vi "pp2_util_paintTableElement.vi"(9 "Color Box":u32(colorbox)=16448250, 10 "Numeric":i32, 11 "Tbl Refnum":refnum<vi>) -> ()   [LabVIEW 2013]
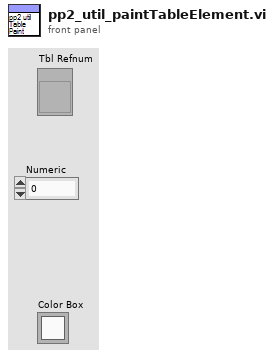
[diagram p1: front panel]
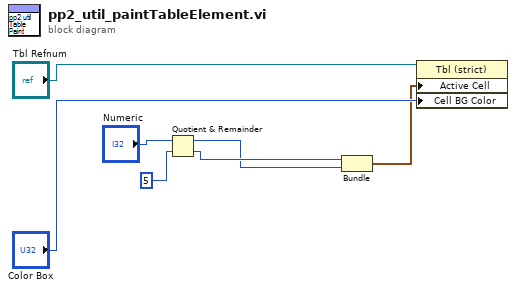
[diagram p0: block diagram]
diagram:
  n1 = Quotient & Remainder(x="Numeric", y=5) -> (x-y*floor(x/y)=w1:i32, floor(x/y)=w2:i32)
  n2 = Bundle(w2, w1) -> (w5:cluster{i32, i32})  [unwired: 1 in]
  n3 = property class="Tbl (strict)"(reference="Tbl Refnum", "Active Cell"=w5, "Cell BG Color"="Color Box") -> ()  [unwired: 1 in, 2 out]
